vi "Sondenmodell.Rücklauftemperatur.vi"(8 "Error in":errorcluster, 10 "Vorlauftemperatur Solekreislauf [°C]":dbl, 11 "Sondenmodell in":refnum<data-value>) -> (0 "Error out":errorcluster, 3 "Sondenmodell out":refnum<data-value>)   [LabVIEW 2016, in "Sondenmodell.lvclass"]
uses:
  Sondenmodell.lvclass
  Sondenmodell.lvclass/Sondenmodell.ctl
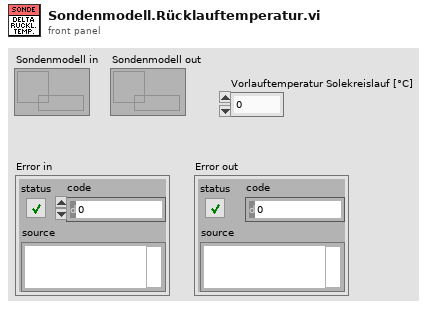
[diagram p1: front panel]
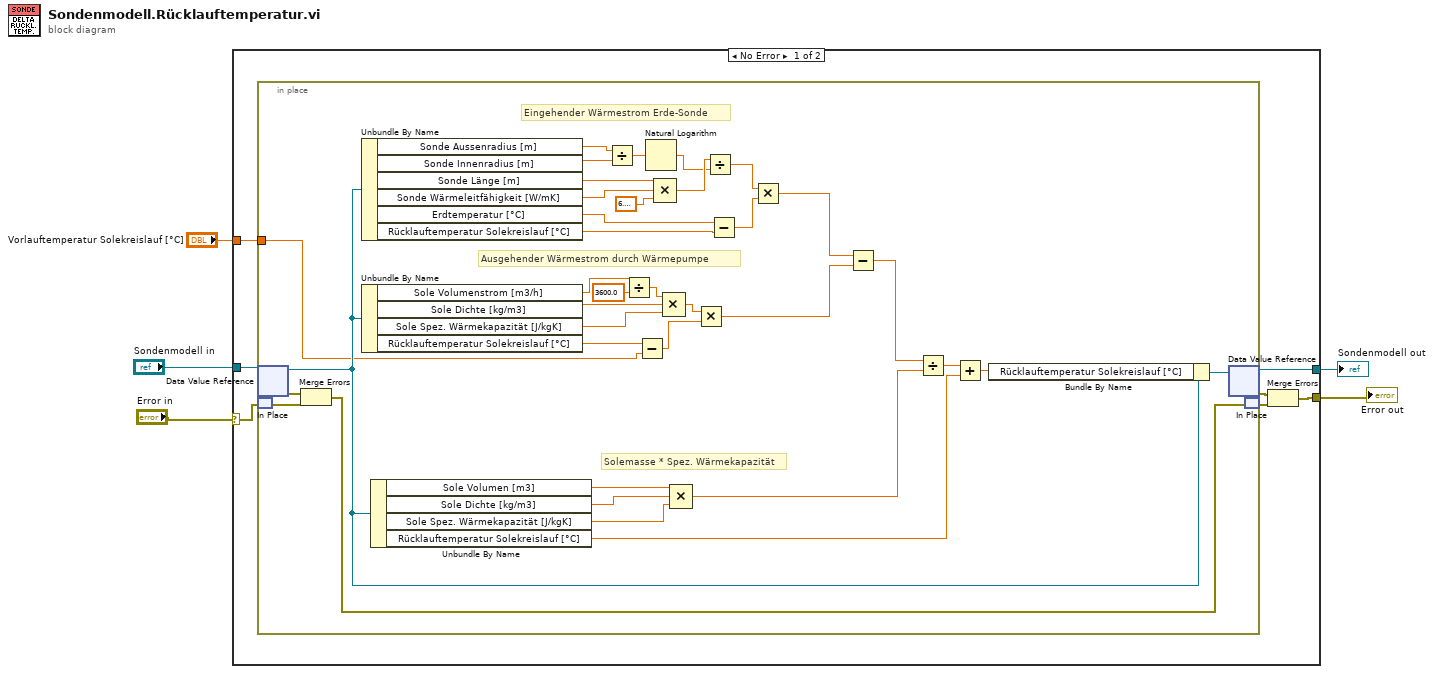
[diagram p0: block diagram]
diagram:
  n1 = case shown="No Error" "Error in" {
    selector: "Error in" -> [w10 w50]
    tunnel: [w9 w49] -> w4
    tunnel: [w8 w50] -> w5
    tunnel: "Sondenmodell in" -> [w7 w49]
    tunnel: "Vorlauftemperatur Solekreislauf [°C]" -> [w6 _]
    frame No Error {
      n2 = in-place {
        in-place-border: w6 -> [w14]
        # "Solemasse * Spez. Wärmekapazität"
        # "Ausgehender Wärmestrom durch Wärmepumpe"
        # "Eingehender Wärmestrom Erde-Sonde"
        n3 = in-place-dvr #1(w7) -> (w21:refnum<class "Sondenmodell.lvclass">, w48:errorcluster)
        n4 = in-place-match #2(w10) -> (w47:errorcluster)
        n5 = Merge Errors(w48, w47) -> (w20:errorcluster)
        n6 = Unbundle By Name(w21) -> ("Sonde Aussenradius [m]"=w34:dbl, "Sonde Innenradius [m]"=w33:dbl, "Sonde Länge [m]"=w31:dbl, "Sonde Wärmeleitfähigkeit [W/mK]"=w30:dbl, "Erdtemperatur [°C]"=w28:dbl, "Rücklauftemperatur Solekreislauf [°C]"=w13:dbl)
        n7 = Unbundle By Name(w21) -> ("Sole Volumenstrom [m3/h]"=w17:dbl, "Sole Dichte [kg/m3]"=w36:dbl, "Sole Spez. Wärmekapazität [J/kgK]"=w35:dbl, "Rücklauftemperatur Solekreislauf [°C]"=w15:dbl)
        n8 = Unbundle By Name(w21) -> ("Sole Volumen [m3]"=w41:dbl, "Sole Dichte [kg/m3]"=w40:dbl, "Sole Spez. Wärmekapazität [J/kgK]"=w39:dbl, "Rücklauftemperatur Solekreislauf [°C]"=w37:dbl)
        n9 = Divide(x=w34, y=w33) -> (x/y=w32:dbl)
        n10 = Divide(x=w17, y=3600.0) -> (x/y=w16:dbl)
        n11 = Subtract(x=w15, y=w14) -> (x-y=w44:dbl)
        n12 = Natural Logarithm(1:w32) -> (0:w26:dbl)
        n13 = Compound Arithmetic op=MULTIPLY(w31, w30, 6.283185307179586) -> (w27:dbl)
        n14 = Compound Arithmetic op=MULTIPLY(w16, w36, w35) -> (w19:dbl)
        n15 = Compound Arithmetic op=MULTIPLY(w41, w40, w39) -> (w38:dbl)
        n16 = Multiply(x=w19, y=w44) -> (x*y=w43:dbl)
        n17 = Divide(x=w27, y=w26) -> (x/y=w25:dbl)
        n18 = Subtract(x=w28, y=w13) -> (x-y=w24:dbl)
        n19 = Multiply(x=w25, y=w24) -> (x*y=w23:dbl)
        n20 = Subtract(x=w23, y=w43) -> (x-y=w46:dbl)
        n21 = Divide(x=w46, y=w38) -> (x/y=w45:dbl)
        n22 = Add(x=w45, y=w37) -> (x+y=w42:dbl)
        n23 = Bundle By Name(cluster=w21, "Rücklauftemperatur Solekreislauf [°C]"=w42) -> (w22:refnum<class "Sondenmodell.lvclass">)
        n24 = in-place-dvr #1(w22) -> (w9:refnum<data-value>, w12:errorcluster)
        n25 = in-place-match #2(w20) -> (w11:errorcluster)
      }
      n26 = Merge Errors(w12, w11) -> (w8:errorcluster)
    }
    frame Error {
    }
  }
  "Sondenmodell out" <- w4
  "Error out" <- w5
